vi "Cleanup Session.vi"(8 "error in":errorcluster, 11 "Plugin in":refnum<class "PXIe4113 DUT Power Control Replacement.lvclass">) -> (0 "error out":errorcluster, 3 "Plugin out":refnum<class "PXIe4113 DUT Power Control Replacement.lvclass">)   [LabVIEW 2026, in "PXIe4113 DUT Power Control Replacement.lvlib" / "PXIe4113 DUT Power Control Replacement.lvclass"]
uses:
  PXIe4113 DUT Power Control Replacement.lvclass
  PXIe4113 DUT Power Control Replacement.lvclass/PXIe4113 DUT Power Control Replacement.ctl
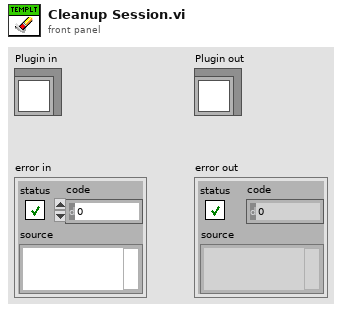
[diagram p1: front panel]
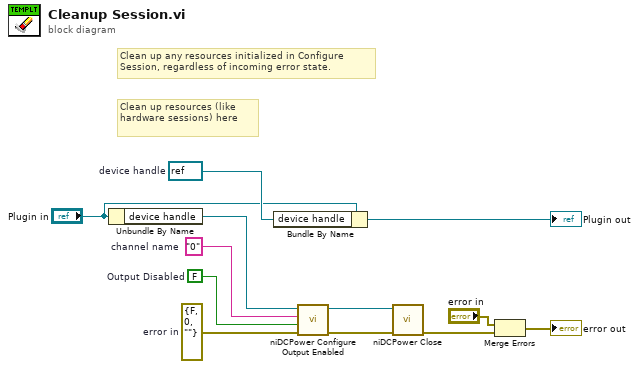
[diagram p0: block diagram]
diagram:
  w6 = refnum<k15> refnum  # device handle
  w9 = errorcluster {"status"=FALSE, "code"=0, "source"=""}  # error in
  w10 = FALSE  # Output Disabled
  w11 = "0"  # channel name
  # "Clean up resources (like hardware sessions) here"
  # "Clean up any resources initialized in Configure Session, regardless of incoming error state."
  n1 = Unbundle By Name("Plugin in") -> ("device handle"=w12:refnum<k15>)
  n2 = Bundle By Name(cluster="Plugin in", "device handle"=w6) -> (→"Plugin out":refnum<class "PXIe4113 DUT Power Control Replacement.lvclass">)
  n3 = call <instrlib>:"niDCPower Configure Output Enabled.vi"("error in (no error)"=w9, "output enabled"=w10, "channel name"=w11, "instrument handle"=w12) -> ("error out"=w7:errorcluster, "instrument handle out"=w8:refnum<k15>)  [unwired: 6 in]
  n4 = call <instrlib>:"niDCPower Close.vi"("error in (no error)"=w7, "instrument handle"=w8) -> ("error out"=w2:errorcluster)  [unwired: 9 in]
  n5 = Merge Errors("error in", w2) -> (→"error out":errorcluster)
